vi "DLP_RecipePrints_XML_Read.vi"(8 "error in (no error)":errorcluster, 11 "Recipe XML File Path":path) -> (0 "error out":errorcluster, 2 "DLPRecipe":T1)   [LabVIEW 2022 SP3]
uses:
  Controls/DLPConfig_RecipePrints.ctl
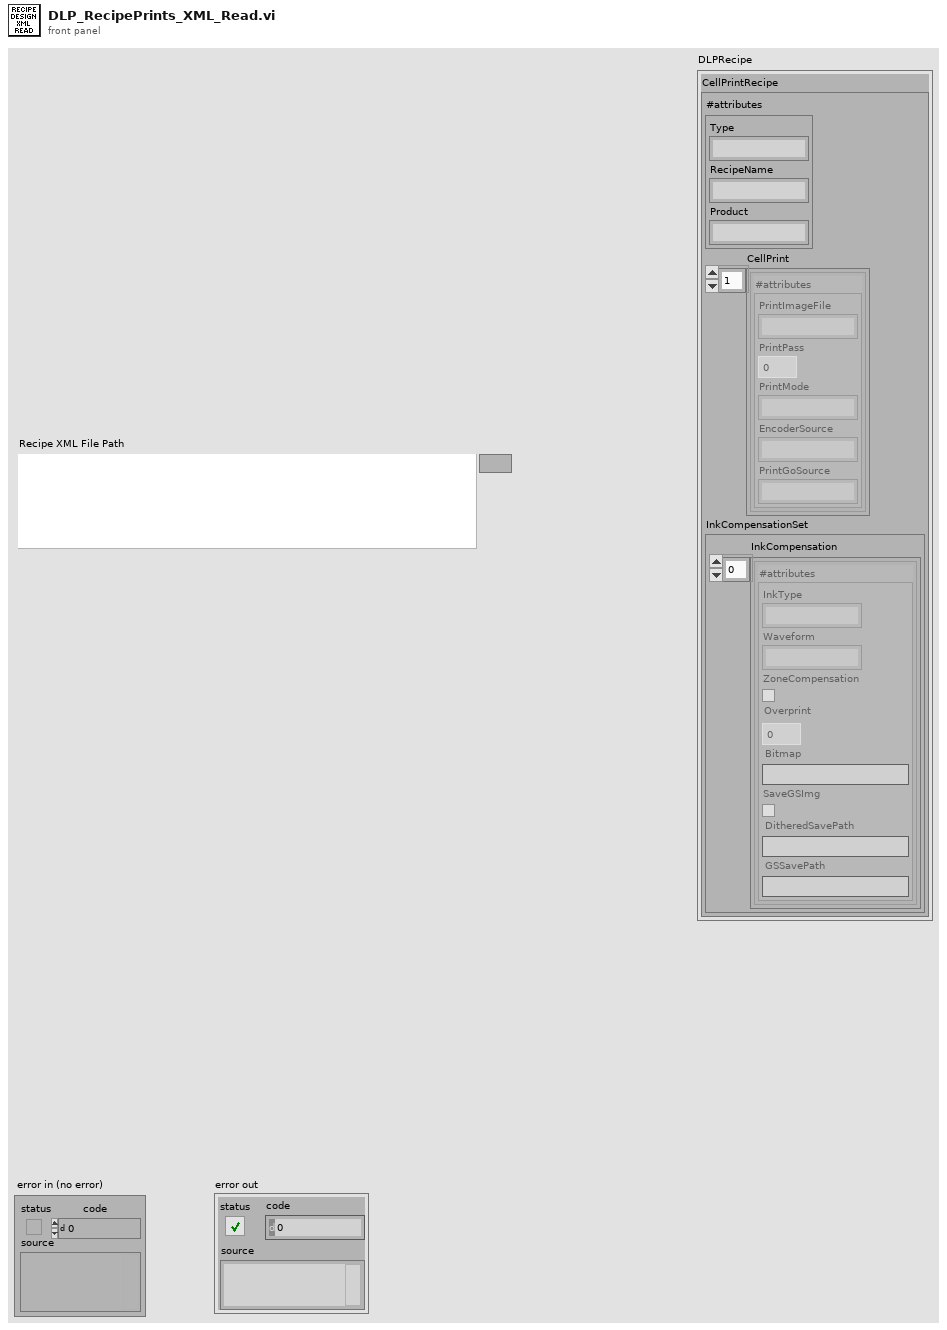
[diagram p1: front panel]
types:
  T1 = typedef "DLPConfig_RecipePrints.ctl" = cluster{"CellPrintRecipe":cluster{"#attributes":cluster{"Type":string, "RecipeName":string, "Product":string}, "CellPrint":cluster{"#attributes":cluster{"PrintImageFile":string, "PrintPass":i32, "PrintMode":string, "EncoderSource":string, "PrintGoSource":string}}[], "InkCompensationSet":cluster{"InkCompensation":cluster{"#attributes":cluster{"InkType":string, "Waveform":string, "ZoneCompensation":bool, "Overprint":dbl, "Bitmap":string, "SaveGSImg":bool, "DitheredSavePath":string, "GSSavePath":string}}[]}}}
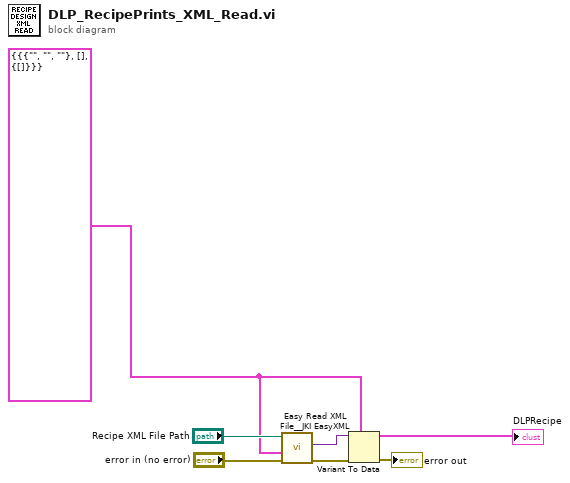
[diagram p0: block diagram]
diagram:
  w1 = T1 {"CellPrintRecipe"={"#attributes"={"Type"="", "RecipeName"="", "Product"=""}, "CellPrint"=[], "InkCompensationSet"={"InkCompensation"=[]}}} ("DLPRecipe")
  n1 = call <vilib>:"Easy Read XML File__JKI EasyXML.vi"("error in (no error)"="error in (no error)", "LabVIEW Data (Type)"=w1, "XML File Path"="Recipe XML File Path") -> ("error out"=w4:errorcluster, "LabVIEW Data"=w5:variant)  [unwired: 6 in, 1 out]
  n2 = Variant To Data(error in=w4, type=w1, Variant=w5) -> (data=→"DLPRecipe":T1, error out=→"error out":errorcluster)
